vi "SetAttributeViInt32_SS-DMod_ListSeq_RF.vi"(7 "AttributeValue":i32 format="%.0g", 8 "error in (no error)":errorcluster {"code" format="%.0x"}, 9 "AttributeID":u32(ring)=1150908 items=["SS_DIGITALMODULATION_ARB_ALC_HOLD "=1150908, "SS_DIGITALMODULATION_ARB_CONTINUOUS_TRIGGER_TYPE "=1150883, "SS_DIGITALMODULATION_ARB_EXTERNAL_TRIGGER_SLOPE "=1150885, "SS_DIGITALMODULATION_ARB_RE_TRIGGER_MODE "=1150888, "SS_DIGITALMODULATION_ARB_RF_BLANKING "=1150909, "SS_DIGITALMODULATION_ARB_RMS_CALCULATION_MODE"=1150892, "SS_DIGITALMODULATION_ARB_SEGMENT_ADVANCE_TRIGGER_TYPE "=1150884, "SS_DIGITALMODULATION_ARB_TRIGGER_SOURCE "=1150881, "SS_DIGITALMODULATION_ARB_TRIGGER_TYPE "=1150882, "SS_LISTSEQUENCER_REPEATITION_MODE "=1150904, "SS_LISTSEQUENCER_SETUP_NUMBER_OF_STEPS "=1150905, "SS_LISTSEQUENCER_SETUP_TRIGGER_TYPE "=1150906, "SS_RFGENERATOR_MODULATION_ANALOG_FORMAT"=1150935, "SS_RFGENERATOR_MODULATION_ANALOG_WAVEFORM_TYPE "=1150936, "SS_RFGENERATOR_MODULATION_TYPE "=1150941, "SS_RFGENERATOR_RADIO_BAND "=1150911, "SS_RFGENERATOR_RADIO_CHANNEL_NUMBER "=1150910], 10 "RepCapIdentifier":string, 11 "instrument handle":refnum<k15>) -> (0 "error out":errorcluster {"code" format="%.0x"}, 3 "instrument handle out":refnum<k15>)   [LabVIEW 2009, in "Keysight XSAn.lvlib"]
doc: "Sets an Int32 attribute from the instrument driver.\nThe following Attributes are supported:\n\nSS_DIGITALMODULATION_ARB_ALC_HOLD \nSS_DIGITALMODULATION_ARB_CONTINUOUS_TRIGGER_TYPE \nSS_DIGITALMODULATION_ARB_EXTERNAL_TRIGGER_SLOPE \nSS_DIGITALMODULATION_ARB_RE_TRIGGER_MODE \nSS_DIGITALMODULATION_ARB_RF_BLANKING \nSS_DIGITALMODULATION_ARB_RMS_CALCULATION_MODE\nSS_DIGITALMODULATION_ARB_SEGMENT_ADVANCE_TRIGGER_TYPE \nSS_DIGITALMODULATION_ARB_TRIGGER_SOURCE \nSS_DIGITALMODULATION_ARB_TRIGGER_TYPE \nSS_LISTSEQUENCER_REPEATITION_MODE \nSS_LISTSEQUENCER_SETUP_NUMBER_OF_STEPS \nSS_LISTSEQUENCER_SETUP_TRIGGER_TYPE \nSS_RFGENERATOR_MODULATION_ANALOG_FORMAT\nSS_RFGENERATOR_MODULATION_ANALOG_WAVEFORM_TYPE \nSS_RFGENERATOR_MODULATION_TYPE \nSS_RFGENERATOR_RADIO_BAND \nSS_RFGENERATOR_RADIO_CHANNEL_NUMBER"
uses:
  <instrlib>/Keysight XSAn/Keysight XSAn.lvlib
  AgXSAn.dll
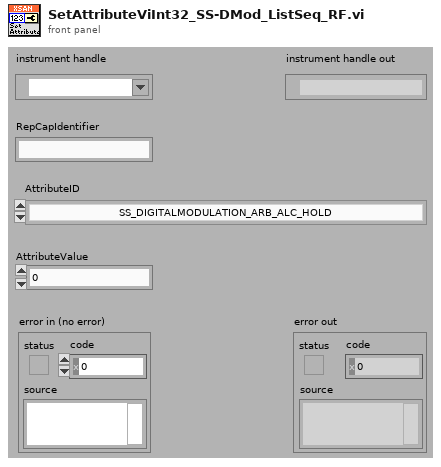
[diagram p1: front panel]
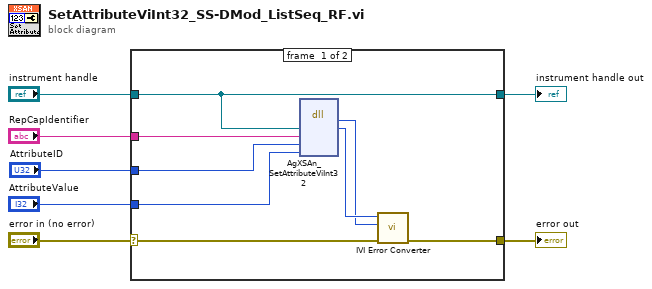
[diagram p0: block diagram]
diagram:
  n1 = case shown="No Error" "error in (no error)" {
    selector: "error in (no error)" -> [w13 w17]
    tunnel: [w12 w17] -> w7
    tunnel: "instrument handle" -> [w8 w16]
    tunnel: "RepCapIdentifier" -> [w11 _]
    tunnel: "AttributeID" -> [w10 _]
    tunnel: "AttributeValue" -> [w9 _]
    tunnel: [w8 w16] -> w2
    frame #0 {
      n2 = dll-call lib="AgXSAn**.dll" fn="AgXSAn_SetAttributeViInt32"("Vi"=w8, "RepCapIdentifier"=w11, "AttributeID"=w10, "AttributeValue"=w9) -> ("return type"=w14:i32, "Vi"=w15:u32)  [unwired: 6 in, 2 out]
      n3 = call <instrlib>:"IVI Error Converter.vi"("error in (no error)"=w13, "IVI error code (0)"=w14, "instrument handle"=w15) -> ("error out"=w12:errorcluster)  [unwired: 7 in, 1 out]
    }
    frame #1 {
    }
  }
  "error out" <- w7
  "instrument handle out" <- w2
